vi "DB Variant To Data_UpdateState2.vi"(0 "XRef":T8, 1 "Old State":T7, 2 "Version":T5) -> (14 "Is Good?":T4, 15 "Reply":T2, 16 "State Out":T1)   [LabVIEW 2010, in "Database Variant To Data.xnode"]
uses:
  <vilib>/addons/database/_DB Variant To Data/Database Variant To Data.xnode
  <vilib>/XNodeSupport/XNodeXNodeRef.ctl
  <vilib>/XNodeSupport/XNodeVariant.ctl
  <vilib>/XNodeSupport/XNodeVersion.ctl
  <vilib>/XNodeSupport/XNodeUShort.ctl
  <vilib>/XNodeSupport/XNodeBool.ctl
  <vilib>/XNodeSupport/XNodeStringArray.ctl
  <vilib>/XNodeSupport/XNodeString.ctl
  <vilib>/addons/database/_DB Variant To Data/DB Variant To Data.ctl
  <vilib>/XNodeSupport/NI_XNodeSupport.lvlib
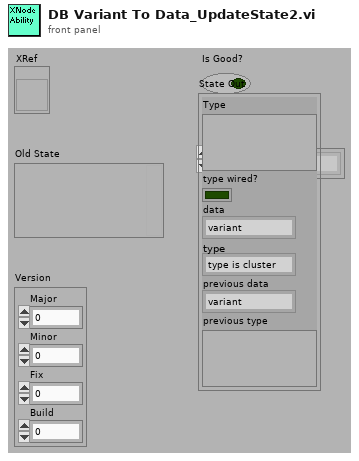
[diagram p1: front panel]
types:
  T1 = typedef "Database Variant To Data.xnode/DB Variant To Data.ctl" = cluster{"Type":variant, "type wired?":bool, "data":enum16{"variant", "variant 1D array", "variant 2D array", "others"}, "type":enum16{"type is cluster", "type is 1D array of scalar type", "type is 1D array of cluster type", "type is 2D array", "type is others", "type is unwired"}, "previous data":enum16{"variant", "variant 1D array", "variant 2D array", "others"}, "previous type":variant}
  T2 = typedef "NI_XNodeSupport.lvlib/XNodeStringArray.ctl" = T3[]
  T3 = typedef "NI_XNodeSupport.lvlib/XNodeString.ctl" = string
  T4 = typedef "NI_XNodeSupport.lvlib/XNodeBool.ctl" = bool
  T5 = typedef "NI_XNodeSupport.lvlib/XNodeVersion.ctl" = cluster{"Major":T6, "Minor":T6, "Fix":T6, "Build":T6}
  T6 = typedef "NI_XNodeSupport.lvlib/XNodeUShort.ctl" = u16
  T7 = typedef "NI_XNodeSupport.lvlib/XNodeVariant.ctl" = variant
  T8 = typedef "NI_XNodeSupport.lvlib/XNodeXNodeRef.ctl" = refnum<vi>
  T9 = enum16{"type is cluster", "type is 1D array of scalar type", "type is 1D array of cluster type", "type is 2D array", "type is others", "type is unwired"}
  T10 = enum16{"variant", "variant 1D array", "variant 2D array", "others"}
  T11 = cluster{"Type":variant, "variant scalar?":bool, "type wired?":bool}
  T12 = cluster{"Type":variant, "type wired?":bool, "data":enum16{"variant", "variant 1D array", "variant 2D array", "others"}, "type":enum16{"type is cluster", "type is 1D array of scalar type", "type is 1D array of cluster type", "type is 2D array", "type is others", "type is unwired"}, "data":enum16{"variant", "variant 1D array", "variant 2D array", "others"}, "Type":variant}
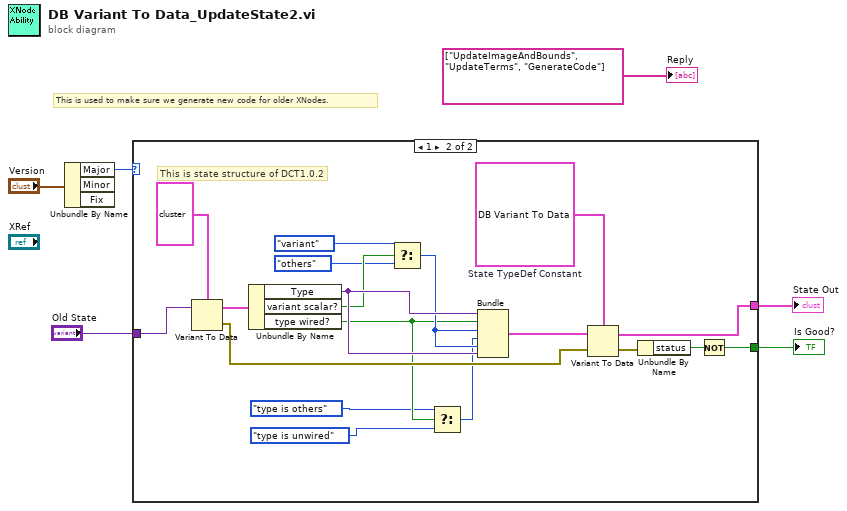
[diagram p0: block diagram]
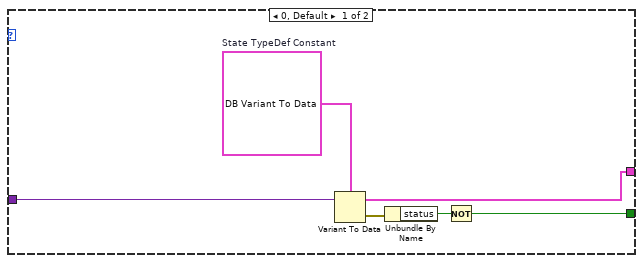
[diagram p2: hidden frame]
diagram:
  # "This is used to make sure we generate new code for older XNodes."
  n1 = Unbundle By Name("Version") -> ("Major"=w4:T6)  [unwired: 2 out]
  n2 = case shown="1" w4 {
    tunnel: "Old State" -> [w8 w15]
    tunnel: [w7 w14] -> w2
    tunnel: [w9 w13] -> w1
    frame 0, Default {
      w11 = T1 {"Type"=variant, "type wired?"=FALSE, "data"=enum."variant", "type"=enum."type is cluster", "previous data"=enum."variant", "previous type"=variant}  # State TypeDef Constant
      n3 = Variant To Data(Variant=w8, type=w11) -> (error out=w12:errorcluster, data=w7:T1)  [unwired: 1 in]
      n4 = Unbundle By Name(w12) -> ("status"=w10:bool)
      n5 = Not(x=w10) -> (.not. x?=w9:bool)
    }
    frame 1 {
      w28 = T1 {"Type"=variant, "type wired?"=FALSE, "data"=enum."variant", "type"=enum."type is cluster", "previous data"=enum."variant", "previous type"=variant}  # State TypeDef Constant
      # "This is state structure of DCT1.0.2"
      n6 = Variant To Data(Variant=w15, type=T11 {"Type"=variant, "variant scalar?"=FALSE, "type wired?"=FALSE}) -> (error out=w30:errorcluster, data=w23:T11)  [unwired: 1 in]
      n7 = Unbundle By Name(w23) -> ("Type"=w27:variant, "variant scalar?"=w25:bool, "type wired?"=w21:bool)
      n8 = Select(t=T10."variant" ("data"), s=w25, f=T10."others" ("data")) -> (s? t:f=w26:T10)
      n9 = Select(t=T9."type is others" ("type"), s=w21, f=T9."type is unwired" ("type")) -> (s? t:f=w18:T9)
      n10 = Bundle("Type"=w27, "type wired?"=w21, "data"=w26, "type"=w18, "data"=w26, "Type"=w27) -> (w29:T12)  [unwired: 1 in]
      n11 = Variant To Data(error in=w30, Variant=w29, type=w28) -> (error out=w31:errorcluster, data=w14:T1)
      n12 = Unbundle By Name(w31) -> ("status"=w24:bool)
      n13 = Not(x=w24) -> (.not. x?=w13:bool)
    }
  }
  "Is Good?" <- w1
  "State Out" <- w2
  "Reply" <- T2 ["UpdateImageAndBounds", "UpdateTerms", "GenerateCode"] ("Reply")
